vi "PhWrite.vi"(5 "PhotInfo64":T2[](array[typedef]) {"flags" max=3 format="%016b"; "rout_chan" step=1; "micro_time" step=1; "mtime" step=1}, 7 "PhotInfo32":T1[](array[typedef]) {"Flags" max=3 format="%016b"; "Routing channel" step=1; "Micro time value" step=1; "Macro time clocks high" step=1; "Macro time clocks low" step=1}, 8 "Error In":errorcluster, 9 "PhFilePath":path, 10 "Module No":i16, 11 "DLL Path":path) -> (0 "error out":errorcluster, 3 "DLL Path":path)   [LabVIEW 2019]
doc: "This VI demonstrates how a PhotInfo-cluster (structure) can be written to a *.ph file in the Becker&Hickl propriety format readable by SPCM.exe\nBoth cluster types (PhotInfo32 and PhotInfo64) are supported.\n\ninfo@becker-hickl.com"
uses:
  SPC_Controls/SPC_PhotInfo64.ctl
  SPC_Controls/SPC_PhotInfo.ctl
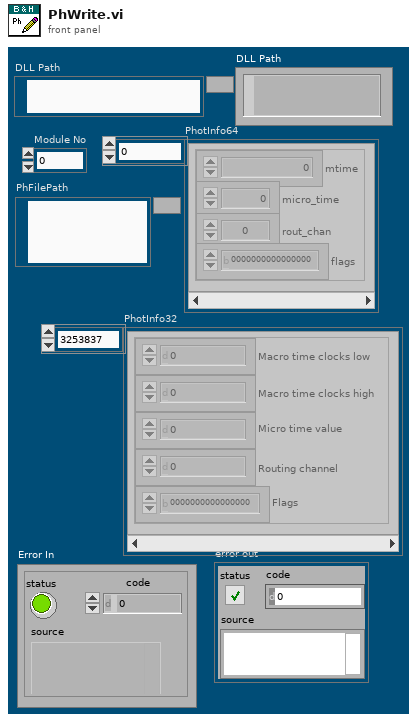
[diagram p1: front panel]
types:
  T1 = typedef "SPC_PhotInfo.ctl" = cluster{"Macro time clocks low":u32, "Macro time clocks high":u32, "Micro time value":u16, "Routing channel":u16, "Flags":u16}
  T2 = typedef "SPC_PhotInfo64.ctl" = cluster{"mtime":u64, "micro_time":u16, "rout_chan":u16, "flags":u16}
  T3 = enum16{"open", "replace", "create", "open or create", "replace or create", "replace or create with confirmation"}
  T4 = enum16{"big-endian, network order", "native, host order", "little-endian"}
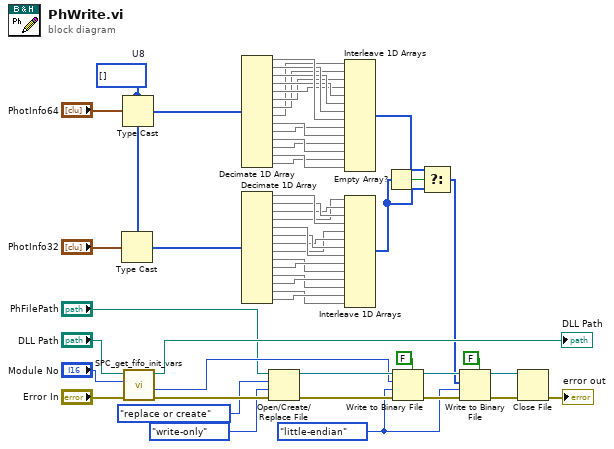
[diagram p0: block diagram]
diagram:
  w22 = u8[] []  # U8
  w46 = T4."little-endian" ("byte order (0:big-endian, network order)")
  n1 = Type Cast(type=w22, x="PhotInfo32") -> (*(type *) &x=w13:u8[])
  n2 = Type Cast(type=w22, x="PhotInfo64") -> (*(type *) &x=w20:u8[])
  n3 = call "SPC_get_fifo_init_vars.vi"("Error In"="Error In", "Module No."="Module No", "DLL Path"="DLL Path") -> ("Error Out"=w55:errorcluster, "spc_header"=w26:u32, "DLL Path"=→"DLL Path":path)  [unwired: 2 in, 4 out]
  n4 = Decimate 1D Array(w20) -> (w40:u8[], w39:u8[], w38:u8[], w37:u8[], w36:u8[], w35:u8[], w34:u8[], w33:u8[], w32:u8[], w31:u8[], w30:u8[], w29:u8[], w28:u8[], w27:u8[])
  n5 = Decimate 1D Array(w13) -> (w9:u8[], w8:u8[], w7:u8[], w6:u8[], w5:u8[], w4:u8[], w3:u8[], w2:u8[], w14:u8[], w15:u8[], w16:u8[], w17:u8[], w18:u8[], w19:u8[])
  n6 = Open/Create/Replace File(file path (use dialog)="PhFilePath", error in=w55, operation (0:open)=T3."replace or create", access (0:read/write)=enum16{"read/write", "read-only", "write-only"}."write-only") -> (refnum out=w49:refnum<file>, error out=w54:errorcluster)  [unwired: 2 in, 1 out]
  n7 = Interleave 1D Arrays(w33, w34, w35, w36, w37, w38, w39, w40, w31, w32, w29, w30, w27, w28) -> (w11:u8[])
  n8 = Interleave 1D Arrays(w6, w7, w8, w9, w2, w3, w4, w5, w15, w14, w17, w16, w19, w18) -> (w12:u8[])
  n9 = Empty Array?(array=w12) -> (empty?=w25:bool)
  n10 = Write to Binary File(file (use dialog)=w49, data=w26, error in=w54, 5:FALSE, 9:w46) -> (refnum out=w48:refnum<file>, error out=w47:errorcluster)  [unwired: 1 in, 1 out]
  n11 = Select(t=w11, s=w25, f=w12) -> (s? t:f=w10:u8[])
  n12 = Write to Binary File(file (use dialog)=w48, data=w10, error in=w47, 5:FALSE ("prepend array or string size? (T)"), 9:w46) -> (refnum out=w50:refnum<file>, error out=w51:errorcluster)  [unwired: 1 in, 1 out]
  n13 = Close File(refnum=w50, error in=w51) -> (error out=→"error out":errorcluster)  [unwired: 1 out]
